vi "serial_clear_reset_wait.vi"(2 "error in (no error)":errorcluster, 3 "VISA Refnum in":refnum<visa-resource-name>) -> (0 "error out":errorcluster, 1 "VISA Refnum out":refnum<visa-resource-name>)   [LabVIEW 2016]
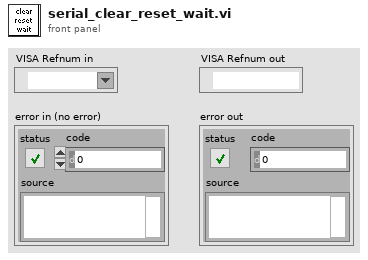
[diagram p1: front panel]
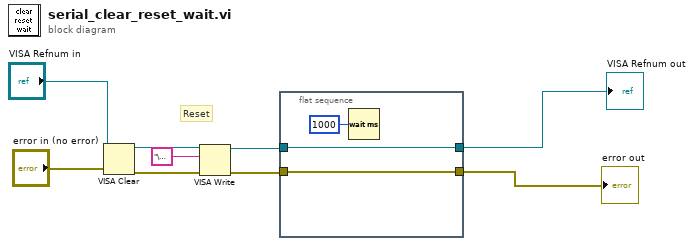
[diagram p0: block diagram]
diagram:
  # "Reset"
  n1 = VISA Clear(VISA resource name="VISA Refnum in", error in (no error)="error in (no error)") -> (VISA resource name out=w3:refnum<visa-resource-name>, error out=w4:errorcluster)
  n2 = VISA Write(VISA resource name=w3, write buffer="\u001b", error in (no error)=w4) -> (VISA resource name out=w8:refnum<visa-resource-name>, error out=w9:errorcluster)  [unwired: 1 out]
  n3 = flat-sequence {
    tunnel: [w12] -> w6
    tunnel: w8 -> [w12]
    tunnel: w9 -> [w10]
    tunnel: [w10] -> w7
    frame #0 {
      n4 = Wait (ms)(milliseconds to wait=u32 1000) -> ()  [unwired: 1 out]
    }
  }
  "error out" <- w7
  "VISA Refnum out" <- w6
